vi "compute path cluster.vi"(2 "path queue":refnum<queue>, 3 "Arrive simultaeously":bool, 4 "error in (no error)":errorcluster, 5 "Step length\n(IMAQ pixels)":dbl, 7 "waypoint queue":refnum<queue>) -> (0 "error out":errorcluster)   [LabVIEW 8.6]
uses:
  Trap cluster.ctl
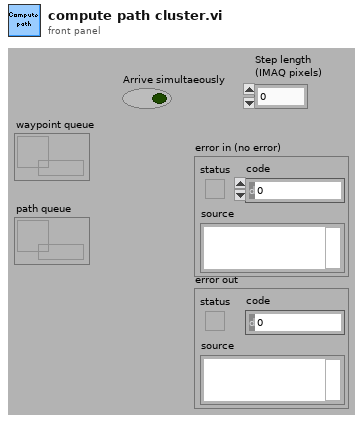
[diagram p1: front panel]
types:
  T1 = typedef "Trap cluster.ctl" = cluster{"X (IMAQ)":dbl[], "Y (IMAQ)":dbl[], "Z":dbl[], "Amplitudes":dbl[], "Trap number":i32[], "ROI number":i32[], "Number of traps":i32, "Group":bool[]}
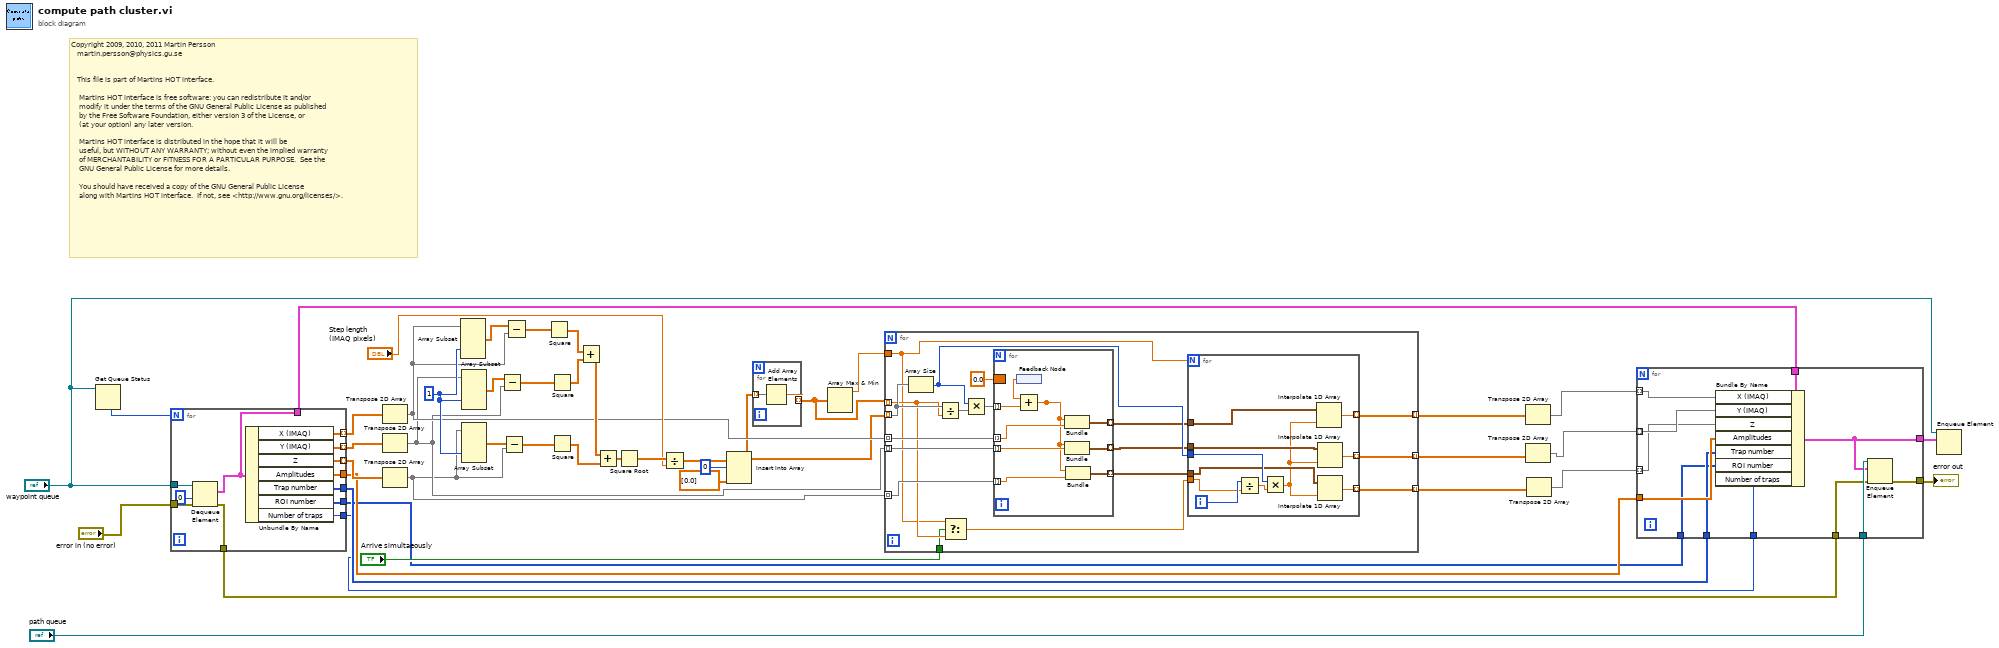
[diagram p0: block diagram]
diagram:
  w42 = 1 ("index")
  # "Copyright 2009, 2010, 2011 Martin Persson \n   martin.persson@physics.gu.se\n\n\n   This file is part of Martins HOT interface.\n\n    Martins HOT interface is free software: you can redistribute it and/or \n    modify it under the terms of the GNU General Public License as published \n    by the Free Software Foundation, either version 3 of the License, or\n    (at your option) any later version.\n\n    Martins HOT interface is distributed in the hope that it will be \n    useful, but WITHOUT ANY WARRANTY; without even the implied warranty\n    of MERCHANTABILITY or FITNESS FOR A PARTICULAR PURPOSE.  See the\n    GNU General Public License for more details.\n\n    You should have received a copy of the GNU General Public License\n    along with Martins HOT interface.  If not, see <http://www.gnu.org/licenses/>."
  n1 = Get Queue Status(queue="waypoint queue") -> (# elements in queue=w3:i32)  [unwired: 2 in, 7 out]
  n2 = for {
    N: w3 -> [_]
    tunnel: [w57] -> w45 mode=indexing
    tunnel: [w56] -> w44 mode=indexing
    tunnel: [w55] -> w43 mode=indexing
    tunnel: [w54] -> w12
    tunnel: [w53] -> w11
    tunnel: [w52] -> w10
    tunnel: [w51] -> w9
    tunnel: [w50] -> w8
    tunnel: "waypoint queue" -> [w49]
    tunnel: "error in (no error)" -> [w48]
    tunnel: [w47] -> w5
    n3 = Dequeue Element(queue=w49, timeout in ms (-1)=0, error in (no error)=w48) -> (element=w50:T1, error out=w47:errorcluster)  [unwired: 2 out]
    n4 = Unbundle By Name(w50) -> ("X (IMAQ)"=w57:dbl[], "Y (IMAQ)"=w56:dbl[], "Z"=w55:dbl[], "Amplitudes"=w54:dbl[], "Trap number"=w53:i32[], "ROI number"=w52:i32[], "Number of traps"=w51:i32)
  }
  n5 = Transpose 2D Array(2D array=w45) -> (transposed array=w26:dbl[][])
  n6 = Transpose 2D Array(2D array=w44) -> (transposed array=w25:dbl[][])
  n7 = Transpose 2D Array(2D array=w43) -> (transposed array=w24:dbl[][])
  n8 = Array Subset(array=w26, index (col)=w42) -> (w31:dbl[][])  [unwired: 3 in]
  n9 = Array Subset(array=w25, index (col)=w42) -> (w30:dbl[][])  [unwired: 3 in]
  n10 = Array Subset(array=w24, index (col)=w42) -> (w29:dbl[][])  [unwired: 3 in]
  n11 = Subtract(x=w30, y=w25) -> (x-y=w40:dbl[][])
  n12 = Subtract(x=w29, y=w24) -> (x-y=w39:dbl[][])
  n13 = Subtract(x=w31, y=w26) -> (x-y=w41:dbl[][])
  n14 = Square(x=w41) -> (x^2=w38:dbl[][])
  n15 = Square(x=w40) -> (x^2=w37:dbl[][])
  n16 = Square(x=w39) -> (x^2=w35:dbl[][])
  n17 = Add(x=w38, y=w37) -> (x+y=w36:dbl[][])
  n18 = Add(x=w36, y=w35) -> (x+y=w34:dbl[][])
  n19 = Square Root(x=w34) -> (sqrt(x)=w33:dbl[][])
  n20 = Divide(x=w33, y="Step length\n(IMAQ pixels)") -> (x/y=w21:dbl[][])
  n21 = Insert Into Array(array=w21, index (col)=0 ("disabled index (col)"), new element=dbl[] [0.0] ("new element/subarray")) -> (w20:dbl[][])  [unwired: 1 in]
  n22 = for {
    tunnel: w20 -> [w59] mode=indexing
    tunnel: [w58] -> w22 mode=indexing
    n23 = Add Array Elements(numeric array=w59) -> (sum=w58:dbl)
  }
  n24 = Array Max & Min(array=w22) -> (max value=w23:dbl)  [unwired: 3 out]
  n25 = for {
    tunnel: w20 -> [w75] mode=indexing
    tunnel: w26 -> [w73] mode=indexing
    tunnel: w25 -> [w72] mode=indexing
    tunnel: w24 -> [w71] mode=indexing
    tunnel: w23 -> [w61]
    tunnel: [w68] -> w18 mode=indexing
    tunnel: w22 -> [w62] mode=indexing
    tunnel: [w65] -> w17 mode=indexing
    tunnel: [w64] -> w16 mode=indexing
    tunnel: "Arrive simultaeously" -> [w60]
    n26 = Array Size(array=w75) -> (size(s)=w70:i32)
    n27 = Divide(x=w75, y=w62) -> (x/y=w77:dbl[])
    n28 = Select(t=w61, s=w60, f=w62) -> (s? t:f=w63:dbl)
    n29 = Multiply(x=w70, y=w77) -> (x*y=w74:dbl[])
    n30 = for {
      tunnel: w74 -> [w97] mode=indexing
      border: 0.0 -> [_]
      tunnel: w73 -> [w95] mode=indexing
      tunnel: w72 -> [w94] mode=indexing
      tunnel: w71 -> [w93] mode=indexing
      tunnel: [w91] -> w69 mode=indexing
      tunnel: [w90] -> w67 mode=indexing
      tunnel: [w89] -> w66 mode=indexing
      n31 = feedback #1() -> (w96:dbl)
      n32 = Add(x=w96, y=w97) -> (x+y=w92:dbl)
      n33 = Bundle(w92, w95) -> (w91:cluster{dbl, dbl})  [unwired: 1 in]
      n34 = Bundle(w92, w94) -> (w90:cluster{dbl, dbl})  [unwired: 1 in]
      n35 = Bundle(w92, w93) -> (w89:cluster{dbl, dbl})  [unwired: 1 in]
    }
    n36 = for {
      N: w61 -> [_]
      tunnel: w63 -> [w87]
      tunnel: w70 -> [w85]
      tunnel: w69 -> [w84]
      tunnel: [w83] -> w68 mode=indexing
      tunnel: w67 -> [w82]
      tunnel: w66 -> [w81]
      tunnel: [w79] -> w65 mode=indexing
      tunnel: [w78] -> w64 mode=indexing
      i -> [w88]
      n37 = Divide(x=w88, y=w87) -> (x/y=w86:dbl)
      n38 = Multiply(x=w85, y=w86) -> (x*y=w80:dbl)
      n39 = Interpolate 1D Array(1:w80, 2:w84) -> (0:w83:dbl)
      n40 = Interpolate 1D Array(1:w80, 2:w82) -> (0:w79:dbl)
      n41 = Interpolate 1D Array(1:w80, 2:w81) -> (0:w78:dbl)
    }
  }
  n42 = Transpose 2D Array(2D array=w18) -> (transposed array=w15:dbl[][])
  n43 = Transpose 2D Array(2D array=w17) -> (transposed array=w14:dbl[][])
  n44 = Transpose 2D Array(2D array=w16) -> (transposed array=w13:dbl[][])
  n45 = for {
    tunnel: w15 -> [w109] mode=indexing
    tunnel: w14 -> [w108] mode=indexing
    tunnel: w13 -> [w107] mode=indexing
    tunnel: w12 -> [w106]
    tunnel: w11 -> [w105]
    tunnel: w10 -> [w104]
    tunnel: w9 -> [w103]
    tunnel: w8 -> [w102]
    tunnel: "path queue" -> [w101]
    tunnel: w5 -> [w100]
    tunnel: [w99] -> w4
    tunnel: [w98] -> w2
    n46 = Bundle By Name(cluster=w102, "X (IMAQ)"=w109, "Y (IMAQ)"=w108, "Z"=w107, "Amplitudes"=w106, "Trap number"=w105, "ROI number"=w104, "Number of traps"=w103) -> (w98:T1)
    n47 = Enqueue Element(queue=w101, element=w98, error in (no error)=w100) -> (error out=w99:errorcluster)  [unwired: 1 in, 2 out]
  }
  "error out" <- w4
  n48 = Enqueue Element(queue="waypoint queue", element=w2) -> ()  [unwired: 2 in, 3 out]
